vi "Begin.vi"() -> (3 "String":string)   [LabVIEW 2018]
panel:
  in  "ОК (ОЗ)":bool
  in  "ОА (ОП)":bool
  out "Лампа":bool=TRUE
  # "Выберите тип индикатора:"
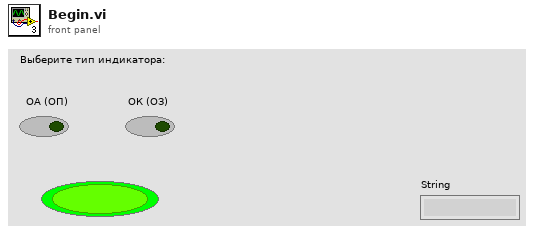
[diagram p1: front panel]
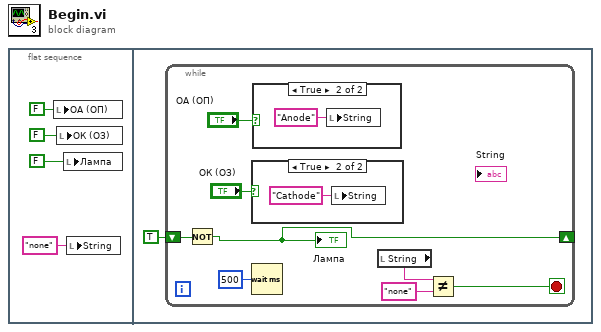
[diagram p0: block diagram]
diagram:
  n1 = flat-sequence {
    frame #0 {
      n2 = local write "ОА (ОП)"(FALSE ("ОА (ОП)")) -> ()
      n3 = local write "ОК (ОЗ)"(FALSE ("ОК (ОЗ)")) -> ()
      n4 = local write "Лампа"(FALSE ("Лампа")) -> ()
      n5 = local write "String"("none" ("String")) -> ()
    }
    frame #1 {
      n6 = while {
        shift-right: [w11] -> _
        shift-left: TRUE -> [w12]
        stop <- w7 stop-if-true
        n7 = Not(x=w12) -> (.not. x?=w11:bool)
        "Лампа" <- w11
        n8 = case shown="True" "ОК (ОЗ)" {
          frame False {
          }
          frame True {
            n9 = local write "String"("Cathode" ("String")) -> ()
          }
        }
        n10 = Wait (ms)(milliseconds to wait=u32 500) -> ()  [unwired: 1 out]
        n11 = case shown="True" "ОА (ОП)" {
          frame False {
          }
          frame True {
            n12 = local write "String"("Anode" ("String")) -> ()
          }
        }
        n13 = local read "String"() -> (w8:string)
        n14 = Not Equal?(x=w8, y="none") -> (x != y?=w7:bool)
      }
    }
  }
